vi "Gen_Daq.vi"(3 "error in":errorcluster, 4 "#DAQ outputs (1-13)":i32, 5 "task/channels in":refnum<k21>) -> (0 "error out":errorcluster, 1 "DaQ_output":dynamicdata(graph), 2 "task out":refnum<k21>)   [LabVIEW 2020]
uses:
  <vilib>/DAQmx/read.llb/DAQmx Read (Analog 1D DBL NChan 1Samp).vi
  <vilib>/DAQmx/miscellaneous.llb/DAQmx Fill In Error Info.vi
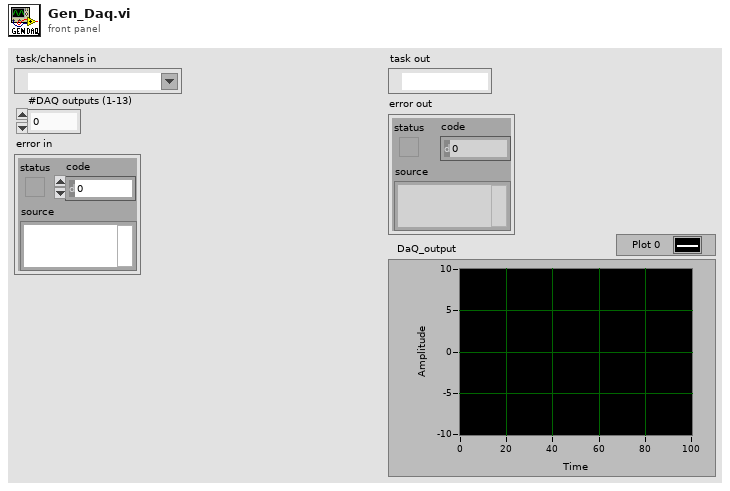
[diagram p1: front panel]
types:
  T1 = cluster{"data[0]":dbl, "data[1]":dbl, "data[2]":dbl}
  T2 = cluster{"data[0]":dbl, "data[1]":dbl, "data[2]":dbl, "data[3]":dbl}
  T3 = cluster{"data[0]":dbl, "data[1]":dbl, "data[2]":dbl, "data[3]":dbl, "data[4]":dbl}
  T4 = cluster{"data[0]":dbl, "data[1]":dbl, "data[2]":dbl, "data[3]":dbl, "data[4]":dbl, "data[5]":dbl}
  T5 = cluster{"data[0]":dbl, "data[1]":dbl, "data[2]":dbl, "data[3]":dbl, "data[4]":dbl, "data[5]":dbl, "data[6]":dbl}
  T6 = cluster{"data[0]":dbl, "data[1]":dbl, "data[2]":dbl, "data[3]":dbl, "data[4]":dbl, "data[5]":dbl, "data[6]":dbl, "data[7]":dbl}
  T7 = cluster{"data[0]":dbl, "data[1]":dbl, "data[2]":dbl, "data[3]":dbl, "data[4]":dbl, "data[5]":dbl, "data[6]":dbl, "data[7]":dbl, "data[8]":dbl}
  T8 = cluster{"data[0]":dbl, "data[1]":dbl, "data[2]":dbl, "data[3]":dbl, "data[4]":dbl, "data[5]":dbl, "data[6]":dbl, "data[7]":dbl, "data[8]":dbl, "data[9]":dbl}
  T9 = cluster{"data[0]":dbl, "data[1]":dbl, "data[2]":dbl, "data[3]":dbl, "data[4]":dbl, "data[5]":dbl, "data[6]":dbl, "data[7]":dbl, "data[8]":dbl, "data[9]":dbl, "data[10]":dbl}
  T10 = cluster{"data[0]":dbl, "data[1]":dbl, "data[2]":dbl, "data[3]":dbl, "data[4]":dbl, "data[5]":dbl, "data[6]":dbl, "data[7]":dbl, "data[8]":dbl, "data[9]":dbl, "data[10]":dbl, "data[11]":dbl}
  T11 = cluster{"data[0]":dbl, "data[1]":dbl, "data[2]":dbl, "data[3]":dbl, "data[4]":dbl, "data[5]":dbl, "data[6]":dbl, "data[7]":dbl, "data[8]":dbl, "data[9]":dbl, "data[10]":dbl, "data[11]":dbl, "data[12]":dbl}
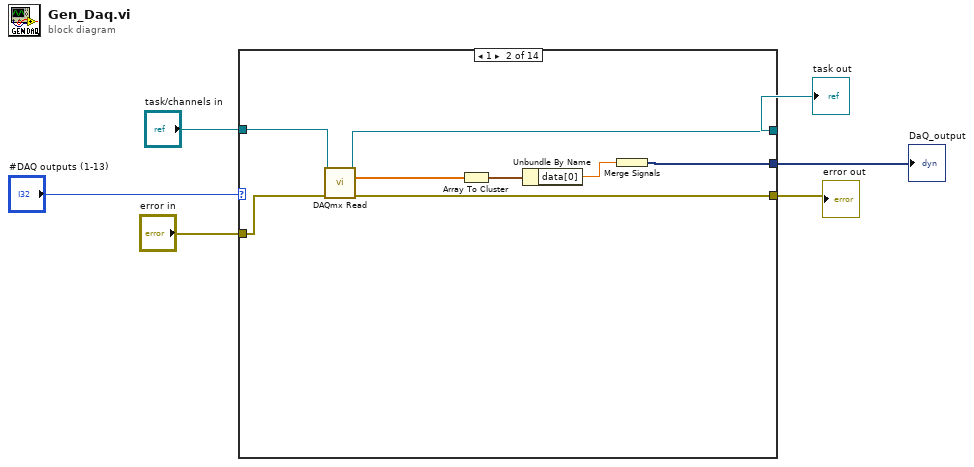
[diagram p0: block diagram]
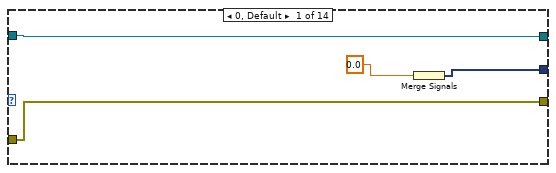
[diagram p2: hidden frame]
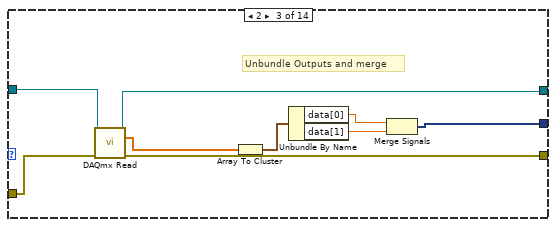
[diagram p3: hidden frame]
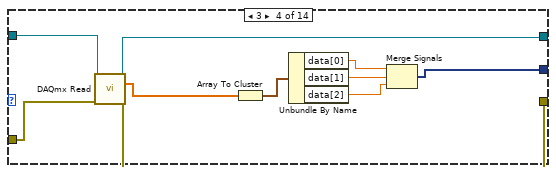
[diagram p4: hidden frame]
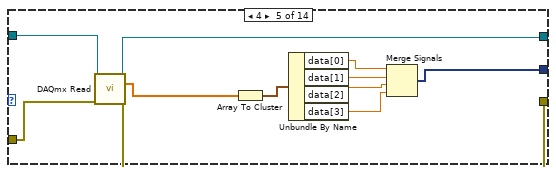
[diagram p5: hidden frame]
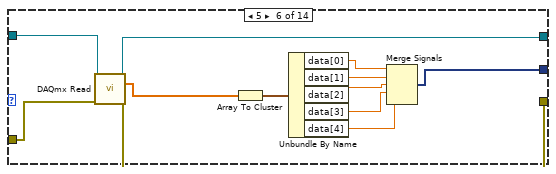
[diagram p6: hidden frame]
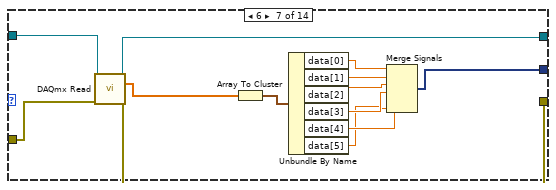
[diagram p7: hidden frame]
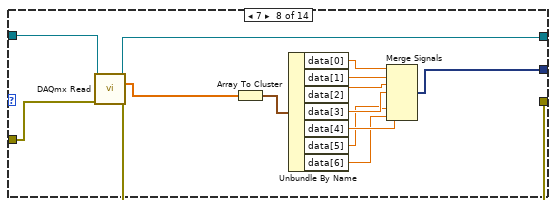
[diagram p8: hidden frame]
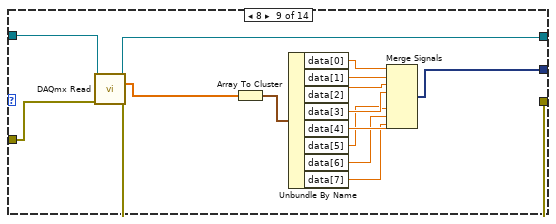
[diagram p9: hidden frame]
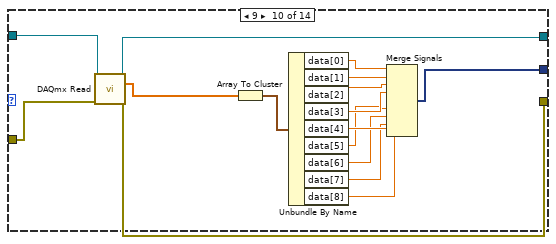
[diagram p10: hidden frame]
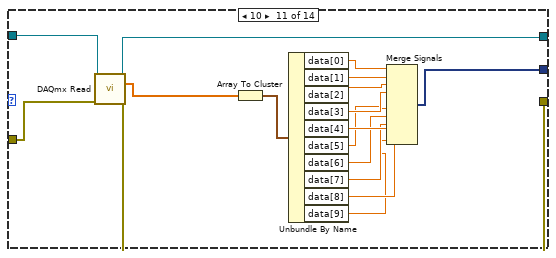
[diagram p11: hidden frame]
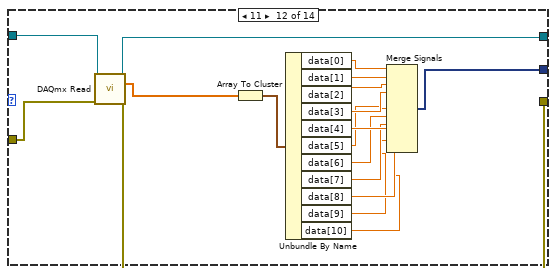
[diagram p12: hidden frame]
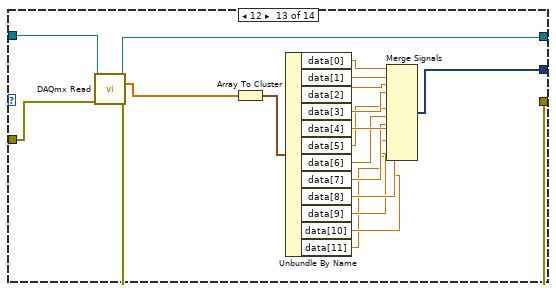
[diagram p13: hidden frame]
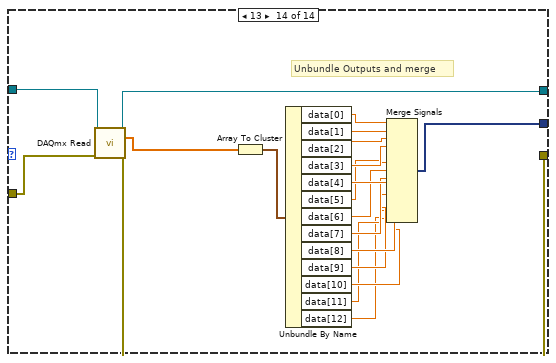
[diagram p14: hidden frame]
diagram:
  n1 = case shown="1" "#DAQ outputs (1-13)" {
    tunnel: "task/channels in" -> [w10 w16 w25 w35 w46 w58 w71 w85 w100 w116 w133 w151 w170 w190]
    tunnel: [w10 w15 w24 w34 w45 w57 w70 w84 w99 w115 w132 w150 w169 w189] -> w5
    tunnel: [w9 w14 w23 w33 w44 w56 w69 w83 w98 w114 w131 w149 w168 w188] -> w4
    tunnel: "error in" -> [w9 w13 w22 w32 w43 w55 w68 w82 w97 w113 w130 w148 w167 w187]
    tunnel: [w7 w11 w20 w30 w41 w53 w66 w80 w95 w111 w128 w146 w165 w185] -> w2
    frame 0, Default {
      n2 = Merge Signals "Merge Signals"(0.0) -> (w7:dynamicdata)
    }
    frame 1 {
      n3 = call-poly <vilib>:"DAQmx Read.vi"("task/channels in"=w16, "error in"=w13) -> ("task out"=w15:refnum<k21>, "data"=w17:dbl[], "error out"=w14:errorcluster)  [unwired: 11 in]
      n4 = Array To Cluster(array=w17) -> (cluster=w18:cluster{"data[0]":dbl})
      n5 = Unbundle By Name(w18) -> ("data[0]"=w12:dbl)
      n6 = Merge Signals "Merge Signals"(w12) -> (w11:dynamicdata)
    }
    frame 2 {
      # "Unbundle Outputs and merge"
      n7 = call-poly <vilib>:"DAQmx Read.vi"("task/channels in"=w25, "error in"=w22) -> ("task out"=w24:refnum<k21>, "data"=w26:dbl[], "error out"=w23:errorcluster)  [unwired: 11 in]
      n8 = Array To Cluster(array=w26) -> (cluster=w27:cluster{"data[0]":dbl, "data[1]":dbl})
      n9 = Unbundle By Name(w27) -> ("data[0]"=w21:dbl, "data[1]"=w19:dbl)
      n10 = Merge Signals "Merge Signals"(w21, w19) -> (w20:dynamicdata)
    }
    frame 3 {
      n11 = call-poly <vilib>:"DAQmx Read.vi"("task/channels in"=w35, "error in"=w32) -> ("task out"=w34:refnum<k21>, "data"=w36:dbl[], "error out"=w33:errorcluster)  [unwired: 11 in]
      n12 = Array To Cluster(array=w36) -> (cluster=w37:T1)
      n13 = Unbundle By Name(w37) -> ("data[0]"=w31:dbl, "data[1]"=w29:dbl, "data[2]"=w28:dbl)
      n14 = Merge Signals "Merge Signals"(w31, w29, w28) -> (w30:dynamicdata)
    }
    frame 4 {
      n15 = call-poly <vilib>:"DAQmx Read.vi"("task/channels in"=w46, "error in"=w43) -> ("task out"=w45:refnum<k21>, "data"=w47:dbl[], "error out"=w44:errorcluster)  [unwired: 11 in]
      n16 = Array To Cluster(array=w47) -> (cluster=w48:T2)
      n17 = Unbundle By Name(w48) -> ("data[0]"=w42:dbl, "data[1]"=w40:dbl, "data[2]"=w39:dbl, "data[3]"=w38:dbl)
      n18 = Merge Signals "Merge Signals"(w42, w40, w39, w38) -> (w41:dynamicdata)
    }
    frame 5 {
      n19 = call-poly <vilib>:"DAQmx Read.vi"("task/channels in"=w58, "error in"=w55) -> ("task out"=w57:refnum<k21>, "data"=w59:dbl[], "error out"=w56:errorcluster)  [unwired: 11 in]
      n20 = Array To Cluster(array=w59) -> (cluster=w60:T3)
      n21 = Unbundle By Name(w60) -> ("data[0]"=w54:dbl, "data[1]"=w52:dbl, "data[2]"=w51:dbl, "data[3]"=w50:dbl, "data[4]"=w49:dbl)
      n22 = Merge Signals "Merge Signals"(w54, w52, w51, w50, w49) -> (w53:dynamicdata)
    }
    frame 6 {
      n23 = call-poly <vilib>:"DAQmx Read.vi"("task/channels in"=w71, "error in"=w68) -> ("task out"=w70:refnum<k21>, "data"=w72:dbl[], "error out"=w69:errorcluster)  [unwired: 11 in]
      n24 = Array To Cluster(array=w72) -> (cluster=w73:T4)
      n25 = Unbundle By Name(w73) -> ("data[0]"=w67:dbl, "data[1]"=w65:dbl, "data[2]"=w64:dbl, "data[3]"=w63:dbl, "data[4]"=w62:dbl, "data[5]"=w61:dbl)
      n26 = Merge Signals "Merge Signals"(w67, w65, w64, w63, w62, w61) -> (w66:dynamicdata)
    }
    frame 7 {
      n27 = call-poly <vilib>:"DAQmx Read.vi"("task/channels in"=w85, "error in"=w82) -> ("task out"=w84:refnum<k21>, "data"=w86:dbl[], "error out"=w83:errorcluster)  [unwired: 11 in]
      n28 = Array To Cluster(array=w86) -> (cluster=w87:T5)
      n29 = Unbundle By Name(w87) -> ("data[0]"=w81:dbl, "data[1]"=w79:dbl, "data[2]"=w78:dbl, "data[3]"=w77:dbl, "data[4]"=w76:dbl, "data[5]"=w75:dbl, "data[6]"=w74:dbl)
      n30 = Merge Signals "Merge Signals"(w81, w79, w78, w77, w76, w75, w74) -> (w80:dynamicdata)
    }
    frame 8 {
      n31 = call-poly <vilib>:"DAQmx Read.vi"("task/channels in"=w100, "error in"=w97) -> ("task out"=w99:refnum<k21>, "data"=w101:dbl[], "error out"=w98:errorcluster)  [unwired: 11 in]
      n32 = Array To Cluster(array=w101) -> (cluster=w102:T6)
      n33 = Unbundle By Name(w102) -> ("data[0]"=w96:dbl, "data[1]"=w94:dbl, "data[2]"=w93:dbl, "data[3]"=w92:dbl, "data[4]"=w91:dbl, "data[5]"=w90:dbl, "data[6]"=w89:dbl, "data[7]"=w88:dbl)
      n34 = Merge Signals "Merge Signals"(w96, w94, w93, w92, w91, w90, w89, w88) -> (w95:dynamicdata)
    }
    frame 9 {
      n35 = call-poly <vilib>:"DAQmx Read.vi"("task/channels in"=w116, "error in"=w113) -> ("task out"=w115:refnum<k21>, "data"=w117:dbl[], "error out"=w114:errorcluster)  [unwired: 11 in]
      n36 = Array To Cluster(array=w117) -> (cluster=w118:T7)
      n37 = Unbundle By Name(w118) -> ("data[0]"=w112:dbl, "data[1]"=w110:dbl, "data[2]"=w109:dbl, "data[3]"=w108:dbl, "data[4]"=w107:dbl, "data[5]"=w106:dbl, "data[6]"=w105:dbl, "data[7]"=w104:dbl, "data[8]"=w103:dbl)
      n38 = Merge Signals "Merge Signals"(w112, w110, w109, w108, w107, w106, w105, w104, w103) -> (w111:dynamicdata)
    }
    frame 10 {
      n39 = call-poly <vilib>:"DAQmx Read.vi"("task/channels in"=w133, "error in"=w130) -> ("task out"=w132:refnum<k21>, "data"=w134:dbl[], "error out"=w131:errorcluster)  [unwired: 11 in]
      n40 = Array To Cluster(array=w134) -> (cluster=w135:T8)
      n41 = Unbundle By Name(w135) -> ("data[0]"=w129:dbl, "data[1]"=w127:dbl, "data[2]"=w126:dbl, "data[3]"=w125:dbl, "data[4]"=w124:dbl, "data[5]"=w123:dbl, "data[6]"=w122:dbl, "data[7]"=w121:dbl, "data[8]"=w120:dbl, "data[9]"=w119:dbl)
      n42 = Merge Signals "Merge Signals"(w129, w127, w126, w125, w124, w123, w122, w121, w120, w119) -> (w128:dynamicdata)
    }
    frame 11 {
      n43 = call-poly <vilib>:"DAQmx Read.vi"("task/channels in"=w151, "error in"=w148) -> ("task out"=w150:refnum<k21>, "data"=w152:dbl[], "error out"=w149:errorcluster)  [unwired: 11 in]
      n44 = Array To Cluster(array=w152) -> (cluster=w153:T9)
      n45 = Unbundle By Name(w153) -> ("data[0]"=w147:dbl, "data[1]"=w145:dbl, "data[2]"=w144:dbl, "data[3]"=w143:dbl, "data[4]"=w142:dbl, "data[5]"=w141:dbl, "data[6]"=w140:dbl, "data[7]"=w139:dbl, "data[8]"=w138:dbl, "data[9]"=w137:dbl, "data[10]"=w136:dbl)
      n46 = Merge Signals "Merge Signals"(w147, w145, w144, w143, w142, w141, w140, w139, w138, w137, w136) -> (w146:dynamicdata)
    }
    frame 12 {
      n47 = call-poly <vilib>:"DAQmx Read.vi"("task/channels in"=w170, "error in"=w167) -> ("task out"=w169:refnum<k21>, "data"=w171:dbl[], "error out"=w168:errorcluster)  [unwired: 11 in]
      n48 = Array To Cluster(array=w171) -> (cluster=w172:T10)
      n49 = Unbundle By Name(w172) -> ("data[0]"=w166:dbl, "data[1]"=w164:dbl, "data[2]"=w163:dbl, "data[3]"=w162:dbl, "data[4]"=w161:dbl, "data[5]"=w160:dbl, "data[6]"=w159:dbl, "data[7]"=w158:dbl, "data[8]"=w157:dbl, "data[9]"=w156:dbl, "data[10]"=w155:dbl, "data[11]"=w154:dbl)
      n50 = Merge Signals "Merge Signals"(w166, w164, w163, w162, w161, w160, w159, w158, w157, w156, w155, w154) -> (w165:dynamicdata)
    }
    frame 13 {
      # "Unbundle Outputs and merge"
      n51 = call-poly <vilib>:"DAQmx Read.vi"("task/channels in"=w190, "error in"=w187) -> ("task out"=w189:refnum<k21>, "data"=w191:dbl[], "error out"=w188:errorcluster)  [unwired: 11 in]
      n52 = Array To Cluster(array=w191) -> (cluster=w192:T11)
      n53 = Unbundle By Name(w192) -> ("data[0]"=w186:dbl, "data[1]"=w184:dbl, "data[2]"=w183:dbl, "data[3]"=w182:dbl, "data[4]"=w181:dbl, "data[5]"=w180:dbl, "data[6]"=w179:dbl, "data[7]"=w178:dbl, "data[8]"=w177:dbl, "data[9]"=w176:dbl, "data[10]"=w175:dbl, "data[11]"=w174:dbl, "data[12]"=w173:dbl)
      n54 = Merge Signals "Merge Signals"(w186, w184, w183, w182, w181, w180, w179, w178, w177, w176, w175, w174, w173) -> (w185:dynamicdata)
    }
  }
  "task out" <- w5
  "error out" <- w4
  "DaQ_output" <- w2
